vi "Andor_live_0.0.2.vi"() -> ()   [LabVIEW 2014]
uses:
  <vilib>/Platform/TimedLoop/XDataNode/timing_clust.ctl
  <vilib>/Platform/TimedLoop/XDataNode/nitl_modes.ctl
  <vilib>/Platform/TimedLoop/XDataNode/wakeup.ctl
  <vilib>/platform/TimedLoop/XDataNode/XDataNode.xnode
  Library Files - Andor and MadCity/Andorlib/atmcd32d.lvlib
  <vilib>/Platform/TimedLoop/XDataNode/XDNodeRunTimeDep.lvlib
panel:
  out "LiveImageArray":u16[](array[numeric])
  out "Total pixel size":i32
  in  "Stop":bool
  in  "Live":bool
  out "Return from Initialize":u32
  out "Detector Y Pixels":i32
  in  "Shut Down":bool
  out "Raising Temperature":i32
  out "Detector X Pixels":i32
  out "Cooling":i32
  out "Return from SetTemperature":u32
  in  "Temperature (deg C)":i32=-70
  in  "Exposure Time (secs)":sgl=0.05 format="%.2f"
  in  "Trigger":u32(ring) items=["Internal", "External"]
  # "TEMPERATURE SET AND MONITORING DONE"
  # "Acquisition Mode: Single Scan\nReadout Mode: Full Vertical Binning\nCools to desired temperature, acquires data and then brings the temperature up to 0 in a controlled way."
  # "Status"
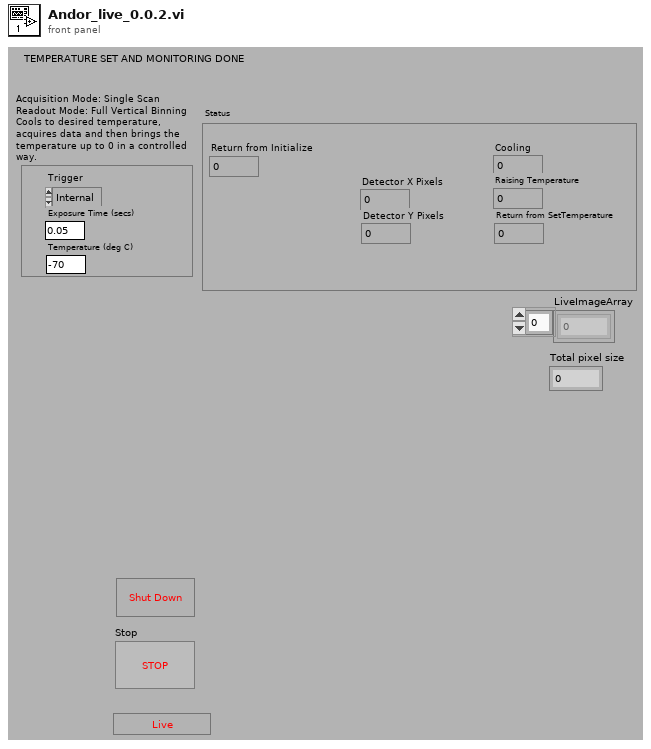
[diagram p1: front panel]
types:
  T1 = typedef "XDNodeRunTimeDep.lvlib/timing_clust.ctl" = cluster{"Expected End [f-1]":u64, "Actual End [f-1]":u64, "Finished Late? [f-1]":bool, "Expected End [i-1]":u64, "Actual End [i-1]":u64, "Finished Late? [i-1]":bool, "Expected Start [i]":u64, "Actual Start [i]":u64, "Expected Start [f]":u64, "Actual Start [f]":u64, "Source Name":string, "Structure Name":string, "Period":i64, "Deadline":i64, "Offset":i64, "Start":i64, "Priority":i32, "Timeout":i32, "Mode":T2, "Wakeup Reason":T3, "Error":errorcluster, "Source Type":string, "Secondary Source Type":string, "Global End Time":u64, "Global Start Time":u64, "Frame Duration":u64, "Iteration Duration":u64, "Assigned CPU":i32, "I/O Scan Engine Mode":u32}
  T2 = typedef "XDNodeRunTimeDep.lvlib/nitl_modes.ctl" = enum32{"No Change", "Process missed periods, maintain original phase", "Discard missed periods, maintain original phase", "Process missed periods, ignore original phase", "Discard missed periods, ignore original phase"}
  T3 = typedef "XDNodeRunTimeDep.lvlib/wakeup.ctl" = enum32{"Normal", "Aborted", "Asynchronous wakeup", "Timing source error", "Timed loop error", "Timeout"}
  T4 = typedef "Image Type" = u32
  T5 = typedef "IMAQ Image.ctl" = refnum<image>
  T6 = enum16{"Full Vertical Binning", "Multi-Track", "Random-Track", "Single-Track", "Image"}
  T7 = enum16{"Reserved (0)", "Single Scan", "Accumulate", "Kinetics", "Fast Kinetics", "Run Till Abort", "Reserved (6)", "Reserved (7)", "Reserved (8)", "Time Delayed Integration"}
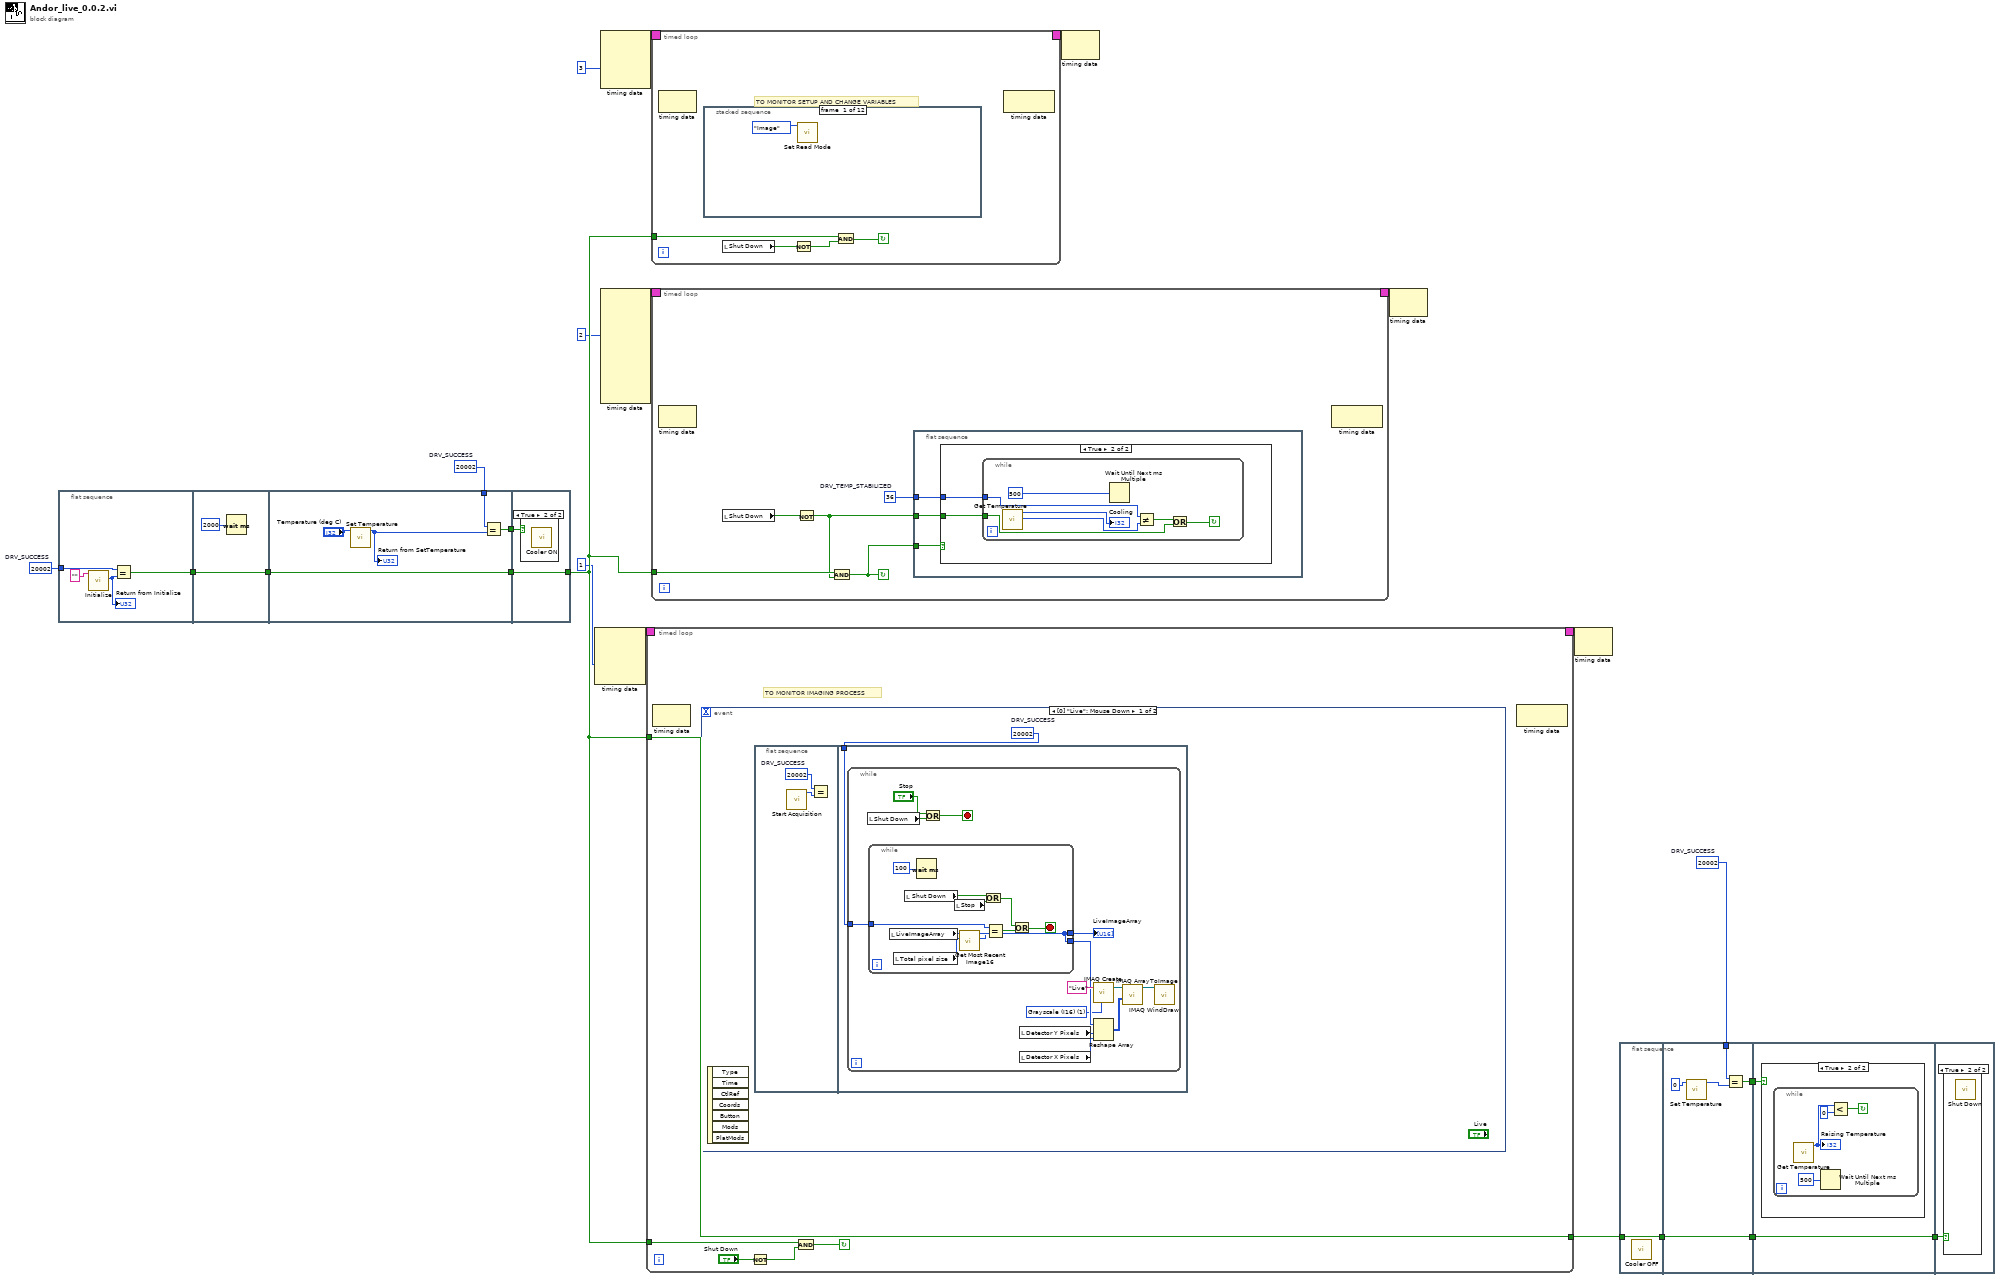
[diagram p0: block diagram]
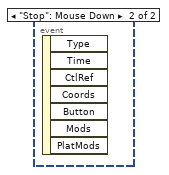
[diagram p6: hidden frame]
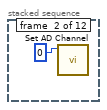
[diagram p7: hidden frame]
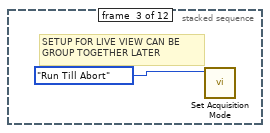
[diagram p8: hidden frame]
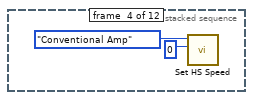
[diagram p9: hidden frame]
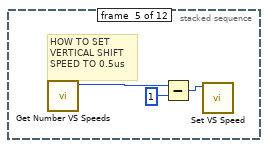
[diagram p10: hidden frame]
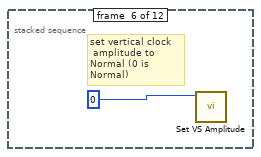
[diagram p11: hidden frame]
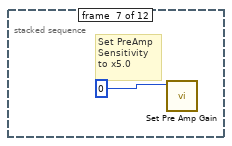
[diagram p12: hidden frame]
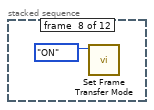
[diagram p13: hidden frame]
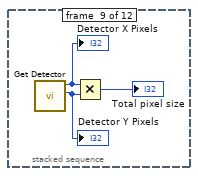
[diagram p14: hidden frame]
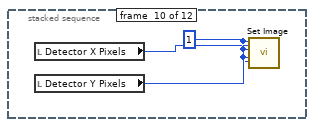
[diagram p15: hidden frame]
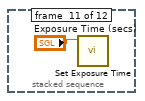
[diagram p16: hidden frame]
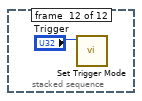
[diagram p17: hidden frame]
diagram:
  w1 = 20002  # DRV_SUCCESS
  w8 = 20002  # DRV_SUCCESS
  w21 = 20002  # DRV_SUCCESS
  n1 = flat-sequence {
    tunnel: w21 -> [w23]
    tunnel: [w24] -> w13
    tunnel: w13 -> [w27]
    tunnel: [w27] -> w4
    tunnel: w4 -> [w33]
    tunnel: [w33] -> w3
    tunnel: [w31] -> w2
    tunnel: w1 -> [w30]
    tunnel: [w35] -> w14
    tunnel: w3 -> [w35]
    tunnel: w2 -> [w34]
    frame #0 {
      n2 = call "Initialize.vi"("dir"="" ("directory (\"\")")) -> ("function return"=w26:u32)  [unwired: 8 in, 2 out]
      "Return from Initialize" <- w26
      n3 = Equal?(x=w23, y=w26) -> (x = y?=w24:bool)
    }
    frame #1 {
      n4 = Wait (ms)(milliseconds to wait=u32 2000) -> ()  [unwired: 1 out]
    }
    frame #2 {
      n5 = call "Set Temperature.vi"("temperature"="Temperature (deg C)") -> ("function return"=w32:u32)  [unwired: 9 in, 1 out]
      "Return from SetTemperature" <- w32
      n6 = Equal?(x=w30, y=w32) -> (x = y?=w31:bool)
    }
    frame #3 {
      n7 = case shown="True" w34 {
        frame False {
        }
        frame True {
          n8 = call "Cooler ON.vi"() -> ()  [unwired: 10 in, 2 out]
        }
      }
    }
  }
  n9 = node-c288(1 ("Priority")) -> (w18:T1)  [unwired: 3 in]
  n10 = node-c288(3 ("Priority")) -> (w20:T1)  [unwired: 3 in]
  n11 = node-c288(2 ("Priority")) -> (w16:T1)  [unwired: 9 in]
  n12 = timed-loop {
    timing: w18 -> [_]
    timing-out: [_] -> w17
    tunnel: [w40] -> w22
    tunnel: w14 -> [w40]
    tunnel: w14 -> [w38]
    stop <- w37 continue-if-true
    # "TO MONITOR IMAGING PROCESS"
    n13 = node-c288() -> ()  [unwired: 1 in, 1 out]
    n14 = event shown="[0] \"Live\": Mouse Down" {
      selector: _ -> [_ _]
      dyn-events: _ -> [_ _]
      timeout: _ -> [_ _]
      event "Live": Mouse Down {
        w41 = 20002  # DRV_SUCCESS
        n15 = event-data() -> ()  [unwired: 1 in, 7 out]
        n16 = flat-sequence {
          tunnel: w41 -> [w44]
          frame #0 {
            w42 = 20002  # DRV_SUCCESS
            n17 = call "Start Acquisition.vi"() -> ("function return"=w43:u32)  [unwired: 10 in, 1 out]
            n18 = Equal?(x=w42, y=w43) -> ()  [unwired: 1 out]
          }
          frame #1 {
            n19 = while {
              tunnel: w44 -> [w45]
              stop <- w49 stop-if-true
              w50 = T4 1 items=["Grayscale (U8)", "Grayscale (I16)", "Grayscale (SGL)", "Complex (CSG)", "RGB (U32)", "HSL (U32)", "RGB (U64)", "Grayscale (U16)"] ("Image Type")
              n20 = local read "Shut Down"() -> (w46:bool)
              n21 = while {
                tunnel: [w67] -> w52
                tunnel: [w67] -> w47
                tunnel: w45 -> [w58]
                stop <- w59 stop-if-true
                n22 = local read "LiveImageArray"() -> (w65:u16[])
                n23 = local read "Total pixel size"() -> (w68:i32)
                n24 = local read "Shut Down"() -> (w63:bool)
                n25 = Wait (ms)(milliseconds to wait=100) -> ()  [unwired: 1 out]
                n26 = local read "Stop"() -> (w66:bool)
                n27 = call "Get Most Recent Image16.vi"("size"=w68, "Array 2"=w65) -> ("function return"=w62:u32, "Array"=w67:u16[])  [unwired: 7 in, 1 out]
                n28 = Or(x=w63, y=w66) -> (x .or. y?=w60:bool)
                n29 = Equal?(x=w58, y=w62) -> (x = y?=w61:bool)
                n30 = Or(x=w60, y=w61) -> (x .or. y?=w59:bool)
              }
              "LiveImageArray" <- w47
              n31 = Or(x="Stop", y=w46) -> (x .or. y?=w49:bool)
              n32 = local read "Detector Y Pixels"() -> (w57:i32)
              n33 = local read "Detector X Pixels"() -> (w56:i32)
              n34 = call "IMAQ Create"("Image Name"="Live", "Image Type"=w50) -> ("New Image"=w55:T5)  [unwired: 3 in, 1 out]
              n35 = Reshape Array(w52, w57, w56) -> (w51:u16[][])
              n36 = call "IMAQ ArrayToImage"("Image Pixels (I16)"=w51, "Image"=w55) -> ("Image Out"=w54:T5)  [unwired: 8 in, 1 out]
              n37 = call "IMAQ WindDraw"("Image"=w54) -> ()  [unwired: 9 in, 2 out]
            }
          }
        }
      }
      event "Stop": Mouse Down {
        n38 = event-data() -> ()  [unwired: 1 in, 7 out]
      }
    }
    n39 = Not(x="Shut Down") -> (.not. x?=w39:bool)
    n40 = And(x=w38, y=w39) -> (x .and. y?=w37:bool)
    n41 = node-c288() -> ()  [unwired: 1 in, 1 out]
  }
  n42 = timed-loop {
    timing: w20 -> [_]
    timing-out: [_] -> w19
    tunnel: w14 -> [w73]
    stop <- w72 continue-if-true
    # "TO MONITOR SETUP AND CHANGE VARIABLES"
    n43 = node-c288() -> ()  [unwired: 1 in, 1 out]
    n44 = stacked-sequence {
      frame #0 {
        n45 = call "Set Read Mode.vi"("mode"=T6."Image") -> ()  [unwired: 9 in, 2 out]
      }
      frame #1 {
        n46 = call "Set AD Channel.vi"("channel"=0) -> ()  [unwired: 9 in, 2 out]
      }
      frame #2 {
        # "SETUP FOR LIVE VIEW CAN BE \nGROUP TOGETHER LATER"
        n47 = call "Set Acquisition Mode.vi"("mode"=T7."Run Till Abort") -> ()  [unwired: 9 in, 2 out]
      }
      frame #3 {
        n48 = call "Set HS Speed.vi"("index"=0, "typ"=enum16{"EM Amp", "Conventional Amp"}."Conventional Amp" ("type")) -> ()  [unwired: 8 in, 2 out]
      }
      frame #4 {
        # "HOW TO SET\nVERTICAL SHIFT\nSPEED TO 0.5us"
        n49 = call "Get Number VS Speeds.vi"() -> ("speeds out"=w82:i32)  [unwired: 9 in, 2 out]
        n50 = Subtract(x=w82, y=1) -> (x-y=w80:i32)
        n51 = call "Set VS Speed.vi"("index"=w80) -> ()  [unwired: 9 in, 2 out]
      }
      frame #5 {
        # "set vertical clock\n amplitude to Normal (0 is Normal)"
        n52 = call "Set VS Amplitude.vi"("index"=0 ("amplitude")) -> ()  [unwired: 9 in, 2 out]
      }
      frame #6 {
        # "Set PreAmp\nSensitivity \nto x5.0"
        n53 = call "Set Pre Amp Gain.vi"("index"=0) -> ()  [unwired: 9 in, 2 out]
      }
      frame #7 {
        n54 = call "Set Frame Transfer Mode.vi"("mode"=enum16{"OFF", "ON"}."ON") -> ()  [unwired: 9 in, 2 out]
      }
      frame #8 {
        n55 = call "Get Detector.vi"() -> ("ypixels out"=w87:i32, "xpixels out"=w88:i32)  [unwired: 8 in, 2 out]
        "Detector Y Pixels" <- w87
        "Detector X Pixels" <- w88
        n56 = Multiply(x=w88, y=w87) -> (x*y=→"Total pixel size":i32)
      }
      frame #9 {
        w89 = 1 ("hbin")
        n57 = local read "Detector X Pixels"() -> (w90:i32)
        n58 = local read "Detector Y Pixels"() -> (w91:i32)
        n59 = call "Set Image.vi"("vend"=w91, "vstart"=w89, "hend"=w90, "hstart"=w89, "vbin"=w89, "hbin"=w89) -> ()  [unwired: 4 in, 2 out]
      }
      frame #10 {
        n60 = call "Set Exposure Time.vi"("time"="Exposure Time (secs)") -> ()  [unwired: 9 in, 2 out]
      }
      frame #11 {
        n61 = call "Set Trigger Mode.vi"("mode"="Trigger") -> ()  [unwired: 9 in, 2 out]
      }
    }
    n62 = local read "Shut Down"() -> (w71:bool)
    n63 = Not(x=w71) -> (.not. x?=w74:bool)
    n64 = And(x=w73, y=w74) -> (x .and. y?=w72:bool)
    n65 = node-c288() -> ()  [unwired: 1 in, 1 out]
  }
  n66 = timed-loop {
    timing: w16 -> [_]
    timing-out: [_] -> w15
    tunnel: w14 -> [w99]
    stop <- w97 continue-if-true
    w100 = 36  # DRV_TEMP_STABILIZED
    n67 = node-c288() -> ()  [unwired: 1 in, 1 out]
    n68 = local read "Shut Down"() -> (w98:bool)
    n69 = Not(x=w98) -> (.not. x?=w96:bool)
    n70 = And(x=w99, y=w96) -> (x .and. y?=w97:bool)
    n71 = flat-sequence {
      tunnel: w100 -> [w103]
      tunnel: w97 -> [w102]
      tunnel: w96 -> [w101]
      frame #0 {
        n72 = case shown="True" w102 {
          tunnel: w103 -> [_ w105]
          tunnel: w101 -> [_ w104]
          frame False {
          }
          frame True {
            n73 = while {
              tunnel: w105 -> [w109]
              tunnel: w104 -> [w106]
              stop <- w107 continue-if-true
              n74 = call "Get Temperature.vi"() -> ("function return"=w110:u32, "temperature out"=→"Cooling":i32)  [unwired: 9 in, 1 out]
              n75 = Wait Until Next ms Multiple(millisecond multiple=u32 500) -> ()  [unwired: 1 out]
              n76 = Not Equal?(x=w109, y=w110) -> (x != y?=w108:bool)
              n77 = Or(x=w108, y=w106) -> (x .or. y?=w107:bool)
            }
          }
        }
      }
    }
    n78 = node-c288() -> ()  [unwired: 1 in, 1 out]
  }
  n79 = node-c288(w19) -> ()  [unwired: 1 out]
  n80 = node-c288(w15) -> ()  [unwired: 1 out]
  n81 = node-c288(w17) -> ()  [unwired: 1 out]
  n82 = flat-sequence {
    tunnel: w22 -> [w115]
    tunnel: [w115] -> w11
    tunnel: w11 -> [w120]
    tunnel: [w120] -> w10
    tunnel: [w118] -> w9
    tunnel: w8 -> [w116]
    tunnel: w10 -> [w122]
    tunnel: [w122] -> w12
    tunnel: w9 -> [w121]
    tunnel: w12 -> [w127]
    frame #0 {
      n83 = call "Cooler OFF.vi"() -> ()  [unwired: 10 in, 2 out]
    }
    frame #1 {
      n84 = call "Set Temperature.vi"("temperature"=0) -> ("function return"=w117:u32)  [unwired: 9 in, 1 out]
      n85 = Equal?(x=w116, y=w117) -> (x = y?=w118:bool)
    }
    frame #2 {
      n86 = case shown="True" w121 {
        frame False {
        }
        frame True {
          n87 = while {
            stop <- w125 continue-if-true
            n88 = call "Get Temperature.vi"() -> ("temperature out"=w124:i32)  [unwired: 9 in, 2 out]
            "Raising Temperature" <- w124
            n89 = Wait Until Next ms Multiple(millisecond multiple=u32 500) -> ()  [unwired: 1 out]
            n90 = Less?(x=w124, y=i16 0) -> (x < y?=w125:bool)
          }
        }
      }
    }
    frame #3 {
      n91 = case shown="True" w127 {
        frame False {
        }
        frame True {
          n92 = call "Shut Down.vi"() -> ()  [unwired: 10 in, 2 out]
        }
      }
    }
  }
